vi "SequentialFileName.vi"(3 "Extention (.dat)":string=".dat", 5 "File Name In":path) -> (0 "Next File Name":path, 2 "File Name With Sequence":path)   [LabVIEW 2019]
uses:
  <vilib>/regexp/Match Regular Expression.xnode
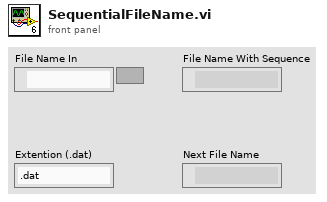
[diagram p1: front panel]
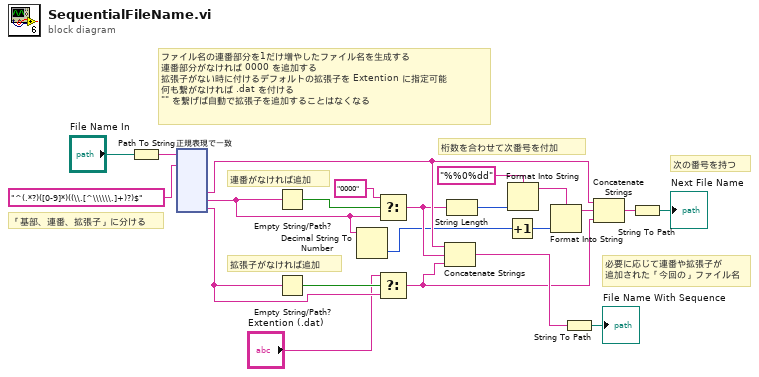
[diagram p0: block diagram]
diagram:
  # "次の番号を持つ"
  # "必要に応じて連番や拡張子が\n追加された「今回の」ファイル名"
  # "拡張子がなければ追加"
  # "桁数を合わせて次番号を付加"
  # "連番がなければ追加"
  # "ファイル名の連番部分を1だけ増やしたファイル名を生成する\n連番部分がなければ 0000 を追加する\n拡張子がない時に付けるデフォルトの拡張子を Extention に指定可能\n何も繋がなければ .dat を付ける\n\"\" を繋げば自動で拡張子を追加することはなくなる"
  # "「基部、連番、拡張子」に分ける"
  n1 = Path To String(path="File Name In") -> (string=w8:string)
  n2 = xnode "正規表現で一致"("input string"=w8, "regular expression"="^(.*?)([0-9]*)((\\.[^\\\\\\.]+)?)$" ("正規表現")) -> ("submatch 1"=w18:string, "submatch 2"=w1:string, "submatch 3"=w3:string)  [unwired: 4 in, 5 out]
  n3 = Empty String/Path?(string/path=w1) -> (empty?=w5:bool)
  n4 = Empty String/Path?(string/path=w3) -> (empty?=w4:bool)
  n5 = Decimal String To Number(string=w1) -> (number=w11:i32)  [unwired: 2 in, 1 out]
  n6 = Select(t="0000", s=w5, f=w1) -> (s? t:f=w12:string)
  n7 = Select(t="Extention (.dat)", s=w4, f=w3) -> (s? t:f=w6:string)
  n8 = Concatenate Strings(w18, w12, w6) -> (w20:string)
  n9 = String Length(string=w12) -> (length=w13:i32)
  n10 = Increment(x=w11) -> (x+1=w15:i32)
  n11 = Format Into String(format string="%%0%dd" ("形式文字列"), w13) -> (resulting string=w16:string)  [unwired: 2 in, 1 out]
  n12 = Format Into String(format string=w16, w15) -> (resulting string=w17:string)  [unwired: 2 in, 1 out]
  n13 = String To Path(string=w20) -> (path=→"File Name With Sequence":path)
  n14 = Concatenate Strings(w18, w17, w6) -> (w19:string)
  n15 = String To Path(string=w19) -> (path=→"Next File Name":path)
